vi "LD50 lead.vi"() -> ()   [LabVIEW 2009]
panel:
  out "Median Lethal dose":dbl[unit]
  in  "weight":dbl[unit]
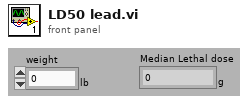
[diagram p1: front panel]
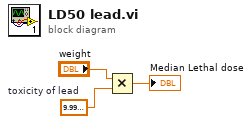
[diagram p0: block diagram]
diagram:
  w2 = dbl[unit] 9.999999999999999e-05  # toxicity of lead
  n1 = Multiply(x="weight", y=w2) -> (x*y=→"Median Lethal dose":dbl[unit])
